vi "圆整至基数的倍数.vi"(1 "base":i32, 2 "input":i32) -> (0 "output":i32)   [LabVIEW 2012]
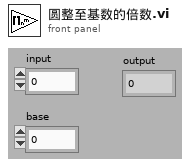
[diagram p1: front panel]
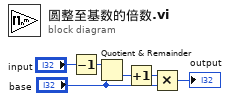
[diagram p0: block diagram]
diagram:
  n1 = Decrement(x="input") -> (x-1=w5:i32)
  n2 = Quotient & Remainder(x=w5, y="base") -> (floor(x/y)=w4:i32)  [unwired: 1 out]
  n3 = Increment(x=w4) -> (x+1=w3:i32)
  n4 = Multiply(x=w3, y="base") -> (x*y=→"output":i32)
